vi "Configure Continuous Acquisition.vi"(8 "error in (no error)":errorcluster, 10 "Enable Continuous Acquisition Mode (T: Enable)":bool=TRUE, 11 "VISA resource name":refnum<visa-resource-name>) -> (0 "error out":errorcluster, 3 "VISA resource name out":refnum<visa-resource-name>)   [LabVIEW 2009, in "Tektronix DPO MSO 2000 4000 Series.lvlib"]
doc: "Configures the oscilloscope to run continuously or to stop after a single acquisition. Run the Initialize VI or the Read Waveform Measurement VI before running this VI."
uses:
  <instrlib>/Tektronix DPO MSO 2000 4000 Series/Tektronix DPO MSO 2000 4000 Series.lvlib
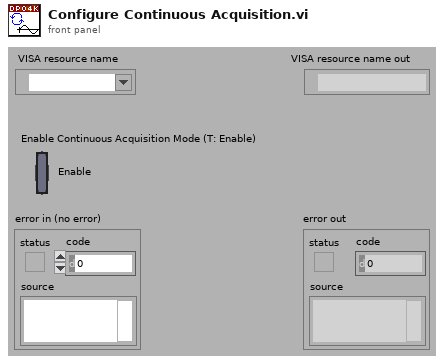
[diagram p1: front panel]
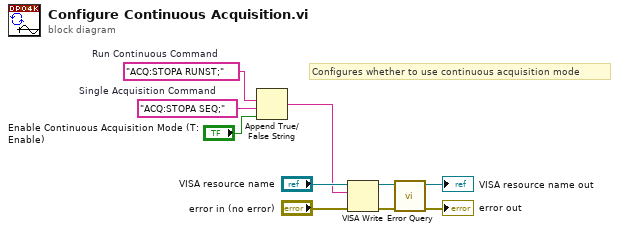
[diagram p0: block diagram]
diagram:
  w3 = "ACQ:STOPA SEQ;"  # Single Acquisition Command
  w4 = "ACQ:STOPA RUNST;"  # Run Continuous Command
  # "Configures whether to use continuous acquisition mode"
  n1 = Append True/False String(1:"Enable Continuous Acquisition Mode (T: Enable)", 2:w3, 3:w4) -> (0:w1:string)  [unwired: 1 in]
  n2 = VISA Write(VISA resource name="VISA resource name", write buffer=w1, error in (no error)="error in (no error)") -> (VISA resource name out=w6:refnum<visa-resource-name>, error out=w5:errorcluster)  [unwired: 1 out]
  n3 = call <instrlib>:"Error Query.vi"("error in (no error)"=w5, "VISA resource name"=w6) -> ("error out"=→"error out":errorcluster, "VISA resource name out"=→"VISA resource name out":refnum<visa-resource-name>)  [unwired: 6 in, 2 out]
